vi "check_infinities&NaNs.vi"(0 "Value":T1 min=-1 max=0.5) -> ()   [LabVIEW 2013]
uses:
  Fast_sequence/sequence slot/DAC_fastseq-offset.ctl
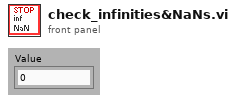
[diagram p1: front panel]
types:
  T1 = typedef "DAC_fastseq-offset.ctl" = sgl
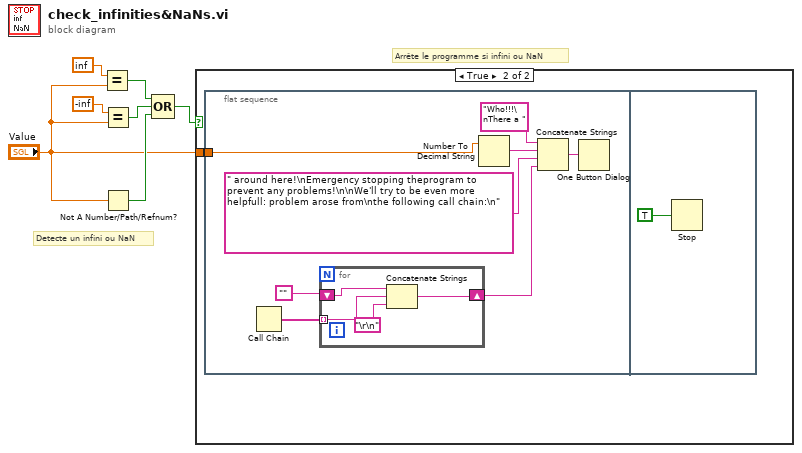
[diagram p0: block diagram]
diagram:
  # "Arrête le programme si infini ou NaN"
  # "Detecte un infini ou NaN"
  n1 = Equal?(x=inf, y="Value") -> (x = y?=w5:bool)
  n2 = Equal?(x=-inf, y="Value") -> (x = y?=w4:bool)
  n3 = Not A Number/Path/Refnum?(number/path/refnum="Value") -> (NaN/Path/Refnum?=w2:bool)
  n4 = Compound Arithmetic op=OR(w5, w4, w2) -> (w3:bool)
  n5 = case shown="True" w3 {
    tunnel: "Value" -> [_ w8]
    frame False {
    }
    frame True {
      n6 = flat-sequence {
        tunnel: w8 -> [w16]
        frame #0 {
          n7 = Call Chain() -> (call chain=w11:string[])
          n8 = for {
            tunnel: w11 -> [w19] mode=indexing
            shift-right: [w20] -> w9
            shift-left: "" -> [w18]
            n9 = Concatenate Strings(w18, w19, "\r\n") -> (w20:string)
          }
          n10 = Number To Decimal String(number=w16) -> (decimal integer string=w15:string)  [unwired: 1 out]
          n11 = Concatenate Strings("Who!!!\nThere a " ("string"), w15, " around here!\nEmergency stopping theprogram to prevent any problems!\n\nWe'll try to be even more helpfull: problem arose from\nthe following call chain:\n" ("string"), w9) -> (w14:string)
          n12 = One Button Dialog(message=w14) -> ()  [unwired: 2 out]
        }
        frame #1 {
          n13 = Stop(stop? (T)=TRUE) -> ()
        }
      }
    }
  }
